vi "CLI_AddParam.vi"(8 "error in (no error)":errorcluster caption="entrée d'erreur (pas d'erreur)", 9 "ParsedParametersIn":cluster{"Name":string, "Value":string}[](array[cluster]), 10 "ParamValue":string, 11 "ParamToAdd":string) -> (0 "Error out":errorcluster, 1 "ParsedParametersOut":cluster{"Name":string, "Value":string}[](array[cluster]))   [LabVIEW 2013]
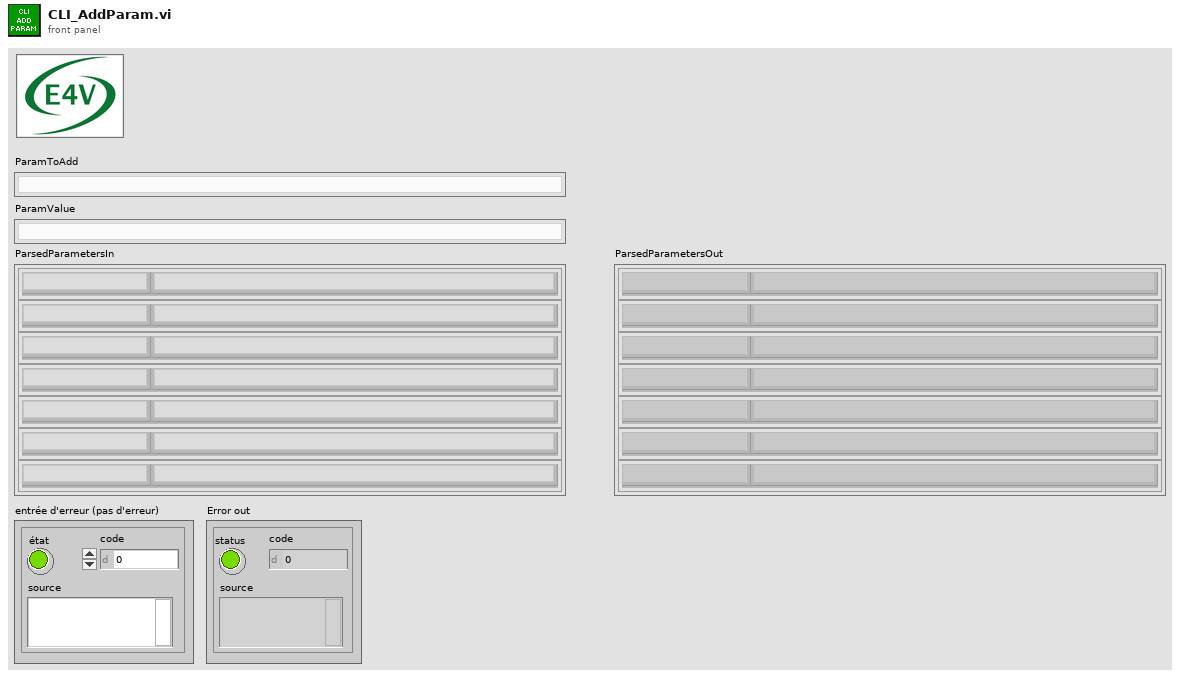
[diagram p1: front panel]
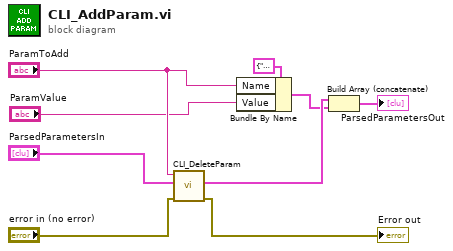
[diagram p0: block diagram]
diagram:
  n1 = call "CLI_DeleteParam.vi"("error in (no error)"="error in (no error)", "ParsedParametersIn"="ParsedParametersIn", "ParamToDelete"="ParamToAdd") -> ("Error out"=→"Error out":errorcluster, "ParsedParametersOut"=w3:cluster{"Name":string, "Value":string}[])  [unwired: 6 in, 1 out]
  n2 = Bundle By Name(cluster=cluster{"Name":string, "Value":string} {"Name"="", "Value"=""} ("cluster d'entrée"), "Name"="ParamToAdd", "Value"="ParamValue") -> (w2:cluster{"Name":string, "Value":string})
  n3 = Build Array (concatenate)(w3, w2) -> (→"ParsedParametersOut":cluster{"Name":string, "Value":string}[])
